vi "PQntuples.vi"(8 "error in (no error)":errorcluster, 10 "res":u32) -> (0 "error out":errorcluster, 3 "PQnTuples":u32)   [LabVIEW 2018, in "libpqlv.lvlib"]
doc: "Returns the number of rows (tuples) in the query result."
uses:
  libpqlv.lvlib
  lib/libpq.dll
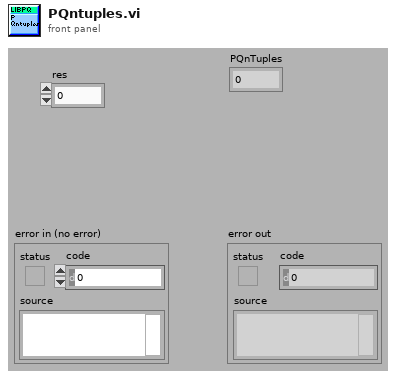
[diagram p1: front panel]
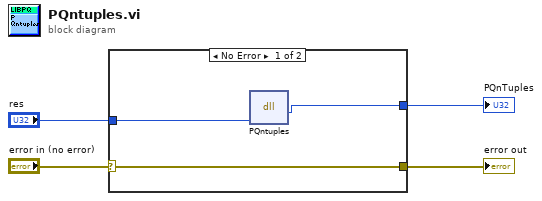
[diagram p0: block diagram]
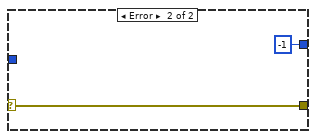
[diagram p2: hidden frame]
diagram:
  n1 = case shown="No Error" "error in (no error)" {
    selector: "error in (no error)" -> [w7 w9]
    tunnel: [w7 w9] -> w3
    tunnel: "res" -> [w6 _]
    tunnel: [w5 -1 ("rows")] -> w1
    frame No Error {
      n2 = dll-call lib="D:/Users/erics/Documents/TC-3/DAQ/PostgreSQL2LabVIEW/libpqlv/lib/libpq.*" fn="PQntuples"("res"=w6) -> ("PQnTuples"=w5:u32)  [unwired: 4 in, 2 out]
    }
    frame Error {
    }
  }
  "PQnTuples" <- w1
  "error out" <- w3
